vi "set pump.vi"(7 "file path":path, 8 "phase":i32, 9 "f":dbl=0.0078125 format="%.4e", 10 "amplitude (volts) in":dbl format="%.2f", 11 "samples":i32=128) -> (2 "amplitude (volts)":dbl format="%.2f", 3 "waveform":sgl[](array[numeric]) format="%.2f", 5 "new file path":path)   [LabVIEW 2010]
uses:
  <vilib>/Utility/file.llb/Read From Spreadsheet File (DBL).vi
  <vilib>/Analysis/NI_AALBase.lvlib
panel:
  # "ticks"
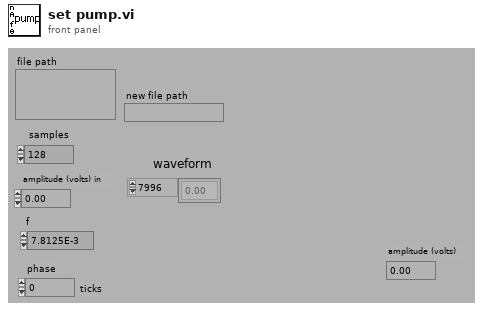
[diagram p1: front panel]
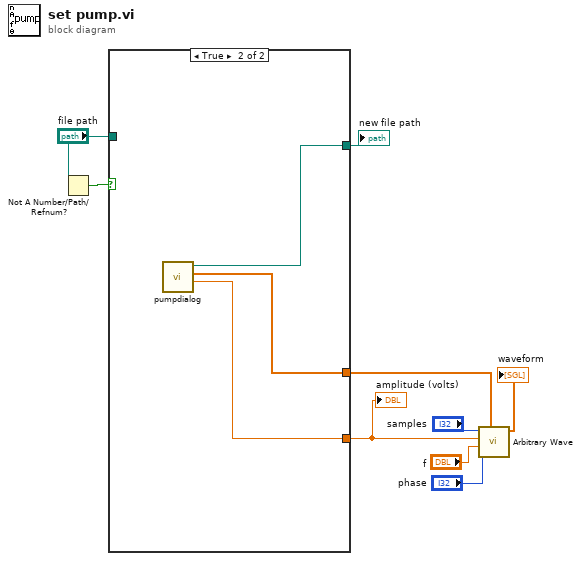
[diagram p0: block diagram]
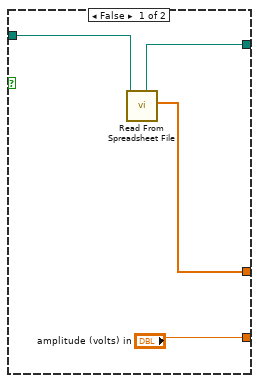
[diagram p2: hidden frame]
diagram:
  n1 = Not A Number/Path/Refnum?(number/path/refnum="file path") -> (NaN/Path/Refnum?=w2:bool)
  n2 = case shown="True" w2 {
    tunnel: [w11 w14] -> w7
    tunnel: "file path" -> [w12 _]
    tunnel: [w10 w16] -> w8
    tunnel: ["amplitude (volts) in" w15] -> w1
    frame False {
      n3 = call-poly <vilib>:"Read From Spreadsheet File.vi"("file path (dialog if empty)"=w12) -> ("first row"=w11:dbl[], "new file path (Not A Path if cancelled)"=w10:path)  [unwired: 6 in, 3 out]
    }
    frame True {
      n4 = call "pumpdialog.vi"() -> ("amplitude (volts)"=w15:dbl, "waveform"=w14:sgl[], "new file path"=w16:path)  [unwired: 9 in]
    }
  }
  "new file path" <- w8
  "amplitude (volts)" <- w1
  n5 = call <vilib>:"Arbitrary Wave.vi"("Wave Table"=w7, "phase in"="phase", "frequency"="f", "amplitude"=w1, "samples"="samples") -> ("arbitrary wave"=→"waveform":dbl[])  [unwired: 2 in, 2 out]
